vi "SequenceIndexToCluster.vi"(11 "SequenceIndex":refnum<class "SequenceIndex.lvclass">) -> (3 "SequenceIndexCluster":cluster{"SequenceIndexName":string, "Steps":u32})   [LabVIEW 2012, in "VariableManagerAPI.lvlib"]
uses:
  VariableManagerAPI.lvlib
  SequenceIndex/SequenceIndex.lvclass
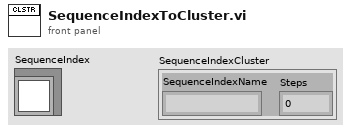
[diagram p1: front panel]
types:
  T1 = cluster{"Accessors:SequenceIndexName":string, "Accessors:Steps":u32}
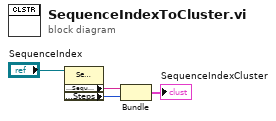
[diagram p0: block diagram]
diagram:
  n1 = property class="SequenceIndex.lvclass"(reference="SequenceIndex") -> ("Accessors:SequenceIndexName"=w3:string, "Accessors:Steps"=w2:u32)  [unwired: 1 in, 2 out]
  n2 = Bundle("Accessors:SequenceIndexName"=w3, "Accessors:Steps"=w2) -> (→"SequenceIndexCluster":T1)  [unwired: 1 in]
